vi "Stop Write Cycle.vi"(11 "error in":errorcluster, 13 "FPGA":T1, 14 "Log (T)":bool=TRUE) -> (15 "error out":errorcluster)   [LabVIEW 2017, in "Host SRL.lvlib"]
uses:
  Host SRL.lvlib
  Type Defs/WSVCAP SHL FPGA Enum.ctl
  Type Defs/WSVCAP SHL Function Enum.ctl
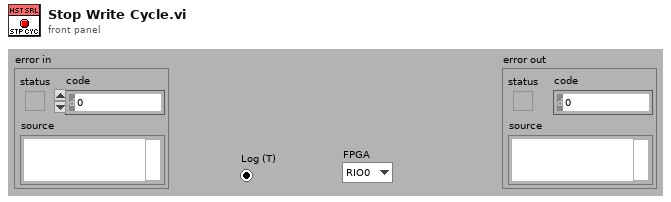
[diagram p1: front panel]
types:
  T1 = typedef "WSVCAP SHL FPGA Enum.ctl" = enum16{"RIO0", "RIO1"}
  T2 = typedef "WSVCAP SHL Function Enum.ctl" = enum16{"Initialize", "Configure I2C", "Configure SRL", "Write I2C", "Read I2C", "Write SRL", "Start SRL Cycle", "Stop SRL Cycle", "Get Status", "Close"}
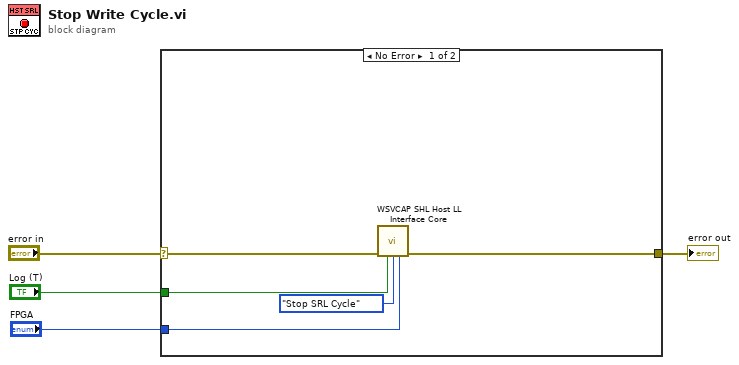
[diagram p0: block diagram]
diagram:
  n1 = case shown="No Error" "error in" {
    selector: "error in" -> [w8 _]
    tunnel: [w7 _] -> w4
    tunnel: "Log (T)" -> [w6 _]
    tunnel: "FPGA" -> [w5 _]
    frame No Error {
      n2 = call "WSVCAP SHL Host LL Interface Core.vi"("error in"=w8, "Log (T)"=w6, "Function"=WSVCAP_SHL_Function_Enum."Stop SRL Cycle", "FPGA"=w5) -> ("error out"=w7:errorcluster)  [unwired: 9 in, 2 out]
    }
    frame Error {
    }
  }
  "error out" <- w4
